vi "solar Create (Application).vi"(8 "error in (no error)":errorcluster, 9 "Menu":refnum<k9>, 10 "VI":refnum<vi>, 11 "Default LVClass":refnum<class "solar.lvclass">) -> (0 "error out":errorcluster, 3 "solar out":refnum<class "solar.lvclass">)   [LabVIEW 2018, in "solar.lvclass"]
doc: "This initializes the SOLAR target references. This assumes that if not targets are defined, this target is the main top level target and performs addition actions to configure the application, launch the splash screen and load the Voyager interface."
uses:
  solar.lvclass
  voyager/solar_voy_ctl Setup.ctl
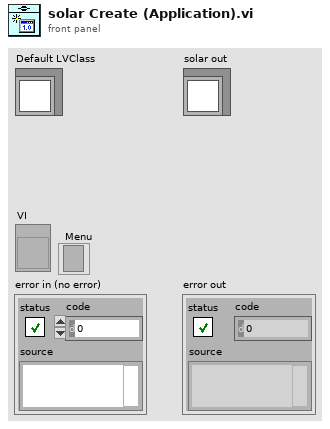
[diagram p1: front panel]
types:
  T1 = typedef "solar_ctl SOLAR Refnum.ctl" = refnum<k1>
  T2 = typedef "solar_ctl SOLAR Global.ctl" = cluster{"Targets":T3[], "AppDir":path, "solar.ini":path, "ConfigsDir":path, "CosmosDir":path, "LogsDir":path, "ExePath":path, "ExeVersion":string, "PartNum":string, "AppSetup":string, "Title":string, "Main.ini":path, "Temp.ini":path, "vSOLAR":string, "Splash.png":string, "SplashWait":i32, "SOLARUE":refnum<user-event>, "VoyagerRefnum":T4, "QTimerRefnum":T5}
  T3 = typedef "solar_ctl Target Global.ctl" = cluster{"Target":string, "Q":refnum<queue>, "UE":refnum<user-event>, "VI":refnum<vi>, "Menu":refnum<k9>, "Data":refnum<data-value>, "Attributes":variant}
  T4 = typedef "solar_voy_ctl Voyager Refnum.ctl" = refnum<k1>
  T5 = typedef "solar_qtimer_ctl Refnum.ctl" = refnum<k1>
  T6 = typedef "solar_voy_ctl Setup.ctl" = cluster{"HEADER":enum8{"LINC", "CCSDS"}, "COSMOS_ROOT":path, "DEFAULT_TARGET":string}
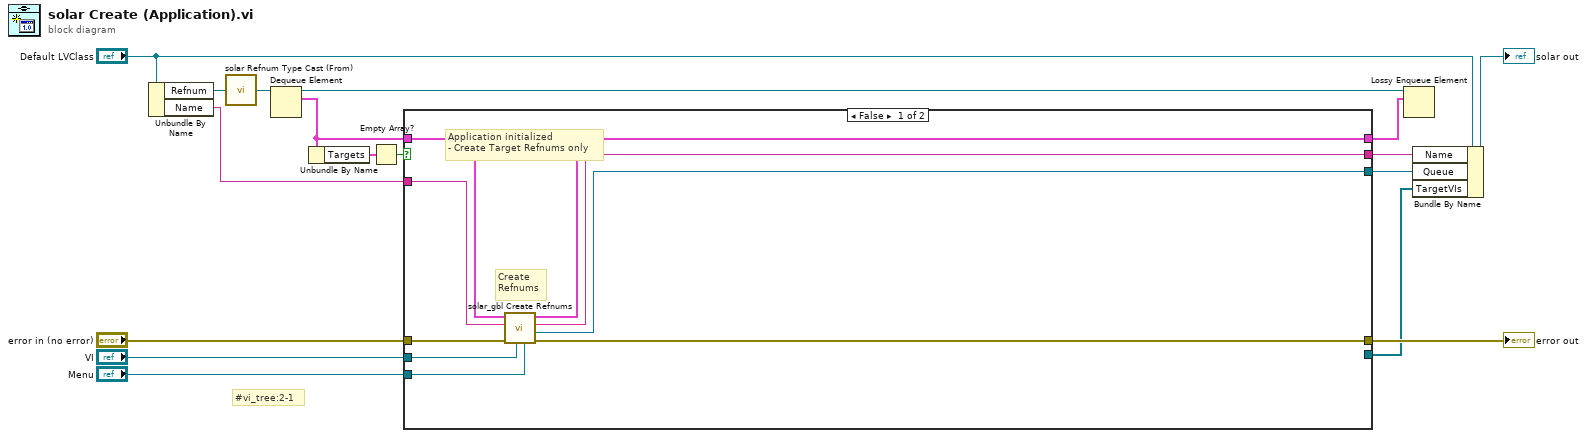
[diagram p0: block diagram]
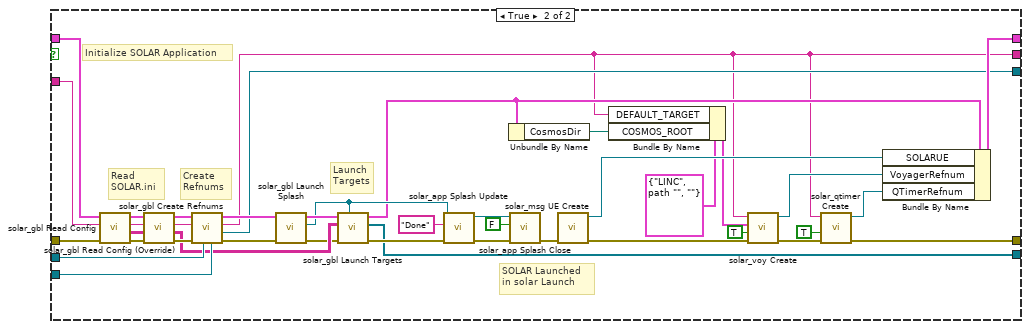
[diagram p2: hidden frame]
diagram:
  # "#vi_tree:2-1"
  n1 = Unbundle By Name("Default LVClass") -> ("Refnum"=w16:T1, "Name"=w8:string)
  n2 = call "solar Refnum Type Cast (From).vi"("Refnum"=w16) -> ("SOLAR"=w15:refnum<queue>)
  n3 = Dequeue Element(queue=w15) -> (queue out=w14:refnum<queue>, element=w12:T2)  [unwired: 2 in, 2 out]
  n4 = Unbundle By Name(w12) -> ("Targets"=w11:T3[])
  n5 = Empty Array?(array=w11) -> (empty?=w5:bool)
  n6 = case shown="False" w5 {
    tunnel: [w23 w44] -> w13
    tunnel: w12 -> [w24 w66]
    tunnel: [w21 w30] -> w9
    tunnel: w8 -> [w22 w34]
    tunnel: "error in (no error)" -> [w26 w65]
    tunnel: [w25 w31] -> w6
    tunnel: "VI" -> [w20 w57]
    tunnel: "Menu" -> [w19 w56]
    tunnel: [w18 w41] -> w2
    tunnel: [_ w27] -> w1
    frame False {
      # "Create\nRefnums"
      # "Application initialized\n- Create Target Refnums only"
      n7 = call "solar_gbl Create Refnums.vi"("Menu"=w19, "VI"=w20, "error in (no error)"=w26, "Name in"=w22, "SOLAR in"=w24) -> ("error out"=w25:errorcluster, "Queue"=w18:refnum<queue>, "Name out"=w21:string, "SOLAR out"=w23:T2)  [unwired: 3 in]
    }
    frame True {
      # "SOLAR Launched\nin solar Launch"
      # "Create\nRefnums"
      # "Read\nSOLAR.ini"
      # "Launch\nTargets"
      # "Initialize SOLAR Application"
      n8 = call "solar_gbl Read Config.vi"("error in (no error)"=w65, "Name in"=w34, "SOLAR in"=w66) -> ("error out"=w64:errorcluster, "Targets"=w61:string[][], "Name out"=w62:string, "SOLAR out"=w63:T2)  [unwired: 5 in]
      n9 = call "solar_gbl Read Config (Override).vi"("error in (no error)"=w64, "Default Targets (name,vi)"=w61, "Name in"=w62, "SOLAR in"=w63) -> ("error out"=w59:errorcluster, "Targets (name,vi)"=w51:string[][], "Name out"=w58:string, "SOLAR out"=w60:T2)  [unwired: 4 in]
      n10 = call "solar_gbl Create Refnums.vi"("Menu"=w56, "VI"=w57, "error in (no error)"=w59, "Name in"=w58, "SOLAR in"=w60) -> ("error out"=w47:errorcluster, "Queue"=w41:refnum<queue>, "Name out"=w30:string, "SOLAR out"=w46:T2)  [unwired: 3 in]
      n11 = call "solar_gbl Launch Splash.vi"("error in (no error)"=w47, "SOLAR in"=w46) -> ("error out"=w45:errorcluster, "Splash VI Refnum"=w50:refnum<vi>, "SOLAR out"=w52:T2)  [unwired: 7 in]
      n12 = call "solar_gbl Launch Targets.vi"("Splash VI Refnum"=w50, "error in (no error)"=w45, "Default Targets (name,vi)"=w51, "SOLAR in"=w52) -> ("error out"=w53:errorcluster, "TargetVIs"=w27:refnum<vi>[], "SOLAR out"=w36:T2)  [unwired: 5 in]
      n13 = call "solar_app Splash Update.vi"("error in (no error)"=w53, "Info"="Done", "Splash VI Refnum in"=w50) -> ("error out"=w55:errorcluster, "Splash VI Refnum out"=w54:refnum<vi>)  [unwired: 7 in]
      n14 = Unbundle By Name(w36) -> ("CosmosDir"=w35:path)
      n15 = call "solar_app Splash Close.vi"("error in (no error)"=w55, "Close Front Panel? (T)"=FALSE, "Splash VI Refnum in"=w54) -> ("error out"=w43:errorcluster)  [unwired: 8 in]
      n16 = call "solar_msg UE Create.vi"("error in (no error)"=w43) -> ("error out"=w40:errorcluster, "UserEvent"=w42:refnum<user-event>)  [unwired: 9 in]
      n17 = Bundle By Name(cluster=T6 {"HEADER"=enum."LINC", "COSMOS_ROOT"=path "", "DEFAULT_TARGET"=""} ("Setup"), "DEFAULT_TARGET"=w30, "COSMOS_ROOT"=w35) -> (w37:T6)
      n18 = call "solar_voy Create.vi"("error in (no error)"=w40, "Create if not found? (T)"=TRUE, "Setup"=w37, "Interface Name"=w30) -> ("error out"=w32:errorcluster, "Voyager Refnum"=w33:T4)  [unwired: 5 in, 1 out]
      n19 = call "solar_qtimer Create.vi"("error in (no error)"=w32, "Create if not found? (T)"=TRUE, "Interface"=w30) -> ("error out"=w31:errorcluster, "QTimer Refnum"=w29:T5)  [unwired: 7 in]
      n20 = Bundle By Name(cluster=w36, "SOLARUE"=w42, "VoyagerRefnum"=w33, "QTimerRefnum"=w29) -> (w44:T2)
    }
  }
  "error out" <- w6
  n21 = Lossy Enqueue Element(queue=w14, element=w13) -> ()  [unwired: 1 in, 4 out]
  n22 = Bundle By Name(cluster="Default LVClass", "Name"=w9, "Queue"=w2, "TargetVIs"=w1) -> (→"solar out":refnum<class "solar.lvclass">)
